vi "Delete Folders and Files (SubVI).vi"(8 "error in (no error)":errorcluster, 11 "selected path":path) -> (0 "error out":errorcluster)   [LabVIEW 2018]
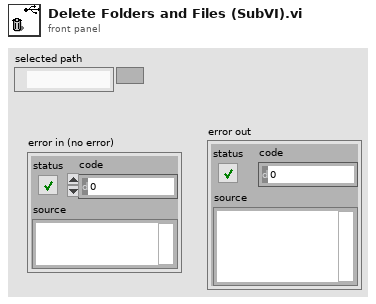
[diagram p1: front panel]
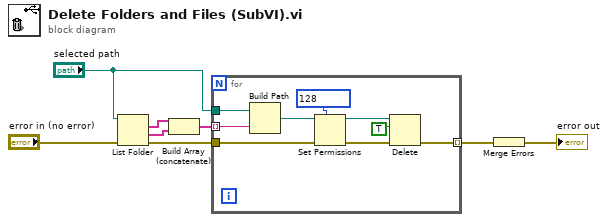
[diagram p0: block diagram]
diagram:
  n1 = List Folder(path="selected path", error in="error in (no error)") -> (filenames=w6:string[], folder names=w5:string[], error out=w4:errorcluster)  [unwired: 2 in, 1 out]
  n2 = Build Array (concatenate)(w6, w5) -> (w8:string[])
  n3 = for {
    tunnel: "selected path" -> [w16]
    tunnel: w8 -> [w15] mode=indexing
    tunnel: w4 -> [w14]
    tunnel: [w9] -> w2 mode=indexing
    n4 = Build Path(base path=w16, name or relative path=w15) -> (appended path=w13:path)
    n5 = Set Permissions(7:i16 128 ("permissions"), 8:w14, 11:w13) -> (0:w10:errorcluster, 3:w11:path)  [unwired: 2 in]
    n6 = Delete(path (use dialog)=w11, entire hierarchy (F)=TRUE, error in=w10) -> (error out=w9:errorcluster)  [unwired: 2 in, 2 out]
  }
  n7 = Merge Errors(w2) -> (→"error out":errorcluster)
